vi "OpenMultipleDevices.vi"() -> ()   [LabVIEW 2013]
uses:
  C:/Code/Apps/Utilities/AG-UC2-UC8/AG-UC2-UC8/Install/Samples/LabVIEW/LabVIEW 2013/CmdLibAgilis.dll
  CmdLibAgilis.dll
panel:
  in  "FwVersion":string
  out "Output:":string
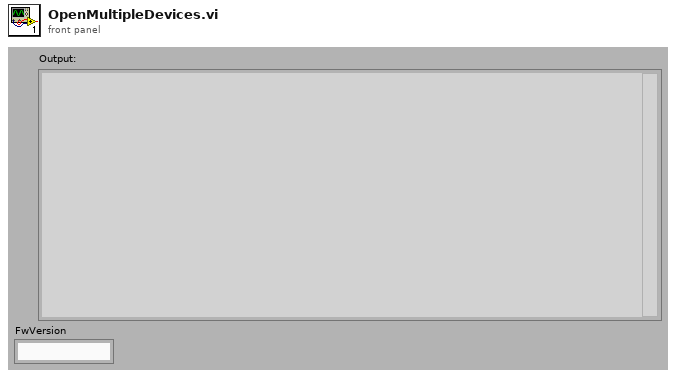
[diagram p1: front panel]
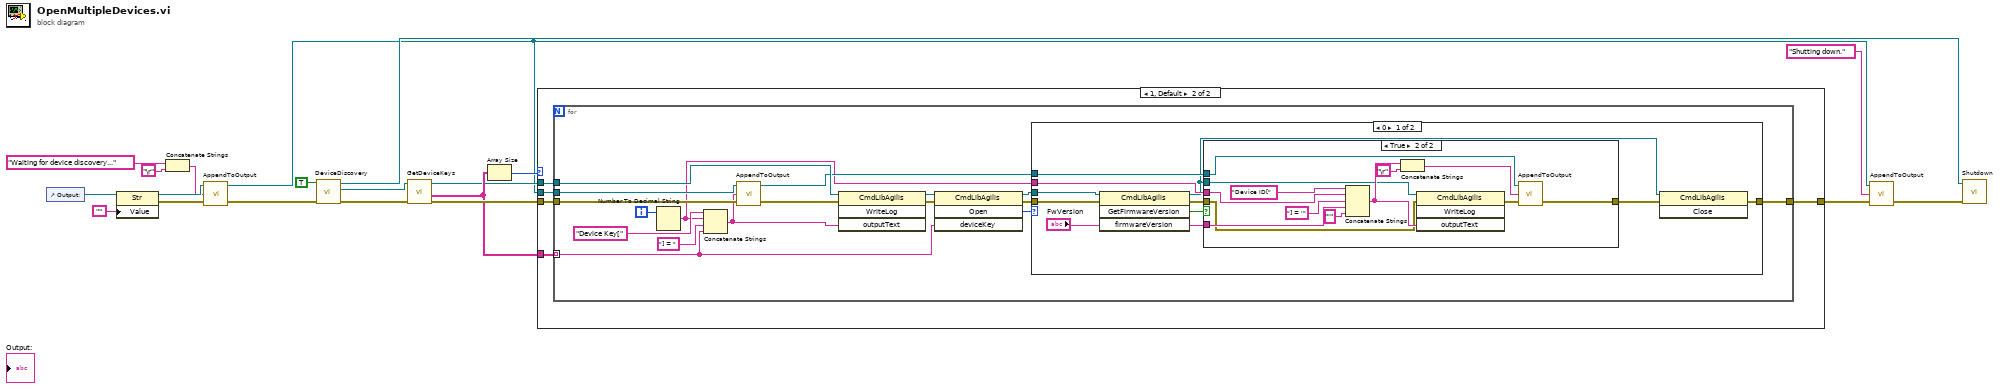
[diagram p0: block diagram]
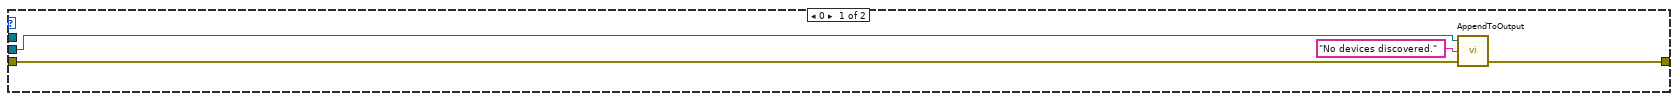
[diagram p2: hidden frame]
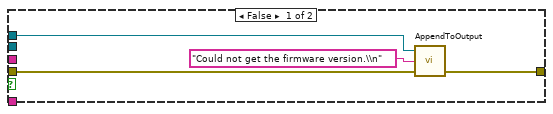
[diagram p3: hidden frame]
diagram:
  n1 = control-ref of="Output:"() -> (w20:refnum<vi>)
  n2 = property class="Str"(reference=w20, "Value"="") -> (reference out=w17:refnum<vi>, error out=w18:errorcluster)  [unwired: 1 in]
  n3 = Concatenate Strings("Waiting for device discovery...", "\r") -> (w7:string)
  n4 = call "AppendToOutput.vi"("error in"=w18, "Input String"=w7, "Output Refnum In"=w17) -> ("error out"=w15:errorcluster, "Output Refnum Out"=w1:refnum<vi>)  [unwired: 1 in]
  n5 = call "DeviceDiscovery.vi"("error in (no error)"=w15, "logging"=TRUE) -> ("error out"=w14:errorcluster, "CmdLib Out"=w13:refnum<k24>, "VCPIOLib Out"=w10:refnum<k24>)  [unwired: 3 in]
  n6 = call "GetDeviceKeys.vi"("error in (no error)"=w14, "CmdLib In"=w13) -> ("error out"=w11:errorcluster, "Device Keys"=w9:string[], "CmdLib Out"=w8:refnum<k24>)  [unwired: 3 in]
  n7 = Array Size(array=w9) -> (size(s)=w12:i32)
  n8 = case shown="1, Default" w12 {
    tunnel: w1 -> [w24 w28]
    tunnel: w11 -> [w23 w27]
    tunnel: w9 -> [_ w29]
    tunnel: w8 -> [_ w26]
    tunnel: [w21 w25] -> w2
    frame 0 {
      n9 = call "AppendToOutput.vi"("error in"=w23, "Input String"="No devices discovered.", "Output Refnum In"=w24) -> ("error out"=w21:errorcluster)  [unwired: 1 in, 1 out]
    }
    frame 1, Default {
      n10 = for {
        tunnel: w29 -> [w38] mode=indexing
        tunnel: w28 -> [w43]
        tunnel: w27 -> [w42]
        tunnel: w26 -> [w39]
        tunnel: [w31] -> w25
        i -> [w46]
        n11 = Number To Decimal String(number=w46) -> (decimal integer string=w30:string)  [unwired: 1 in]
        n12 = Concatenate Strings("Device Key[", w30, "] = ", w38) -> (w41:string)
        n13 = call "AppendToOutput.vi"("error in"=w42, "Input String"=w41, "Output Refnum In"=w43) -> ("error out"=w40:errorcluster, "Output Refnum Out"=w32:refnum<vi>)  [unwired: 1 in]
        n14 = invoke class="CmdLibAgilis" method="WriteLog"(reference=w39, error in=w40, "outputText"=w41) -> (reference out=w37:refnum<k24>, error out=w36:errorcluster)  [unwired: 1 in, 2 out]
        n15 = invoke class="CmdLibAgilis" method="Open"(reference=w37, error in=w36, "deviceKey"=w38) -> (reference out=w34:refnum<k24>, error out=w33:errorcluster, "Open"=w35:i32)  [unwired: 1 in, 1 out]
        n16 = case shown="0" w35 {
          tunnel: w34 -> [w57 _]
          tunnel: w33 -> [w56 w75]
          tunnel: w32 -> [w52 _]
          tunnel: [w50 w75] -> w31
          tunnel: w30 -> [w48 _]
          frame 0 {
            n17 = invoke class="CmdLibAgilis" method="GetFirmwareVersion"(reference=w57, error in=w56, "firmwareVersion"="FwVersion") -> (reference out=w47:refnum<k24>, error out=w53:errorcluster, "GetFirmwareVersion"=w54:bool, "firmwareVersion"=w49:string)  [unwired: 1 in]
            n18 = case shown="True" w54 {
              tunnel: w53 -> [w61 w66]
              tunnel: w52 -> [w60 w69]
              tunnel: [w58 w64] -> w51
              tunnel: w49 -> [_ w72]
              tunnel: w48 -> [_ w71]
              tunnel: w47 -> [_ w63]
              frame False {
                n19 = call "AppendToOutput.vi"("error in"=w61, "Input String"="Could not get the firmware version.\\n" ("firmwareVersion"), "Output Refnum In"=w60) -> ("error out"=w58:errorcluster)  [unwired: 1 in, 1 out]
              }
              frame True {
                n20 = Concatenate Strings("Device ID[", w71, "] = '", w72, "'" ("string")) -> (w68:string)
                n21 = Concatenate Strings(w68, "\r") -> (w67:string)
                n22 = invoke class="CmdLibAgilis" method="WriteLog"(reference=w63, error in=w66, "outputText"=w68) -> (error out=w65:errorcluster)  [unwired: 1 in, 3 out]
                n23 = call "AppendToOutput.vi"("error in"=w65, "Input String"=w67, "Output Refnum In"=w69) -> ("error out"=w64:errorcluster)  [unwired: 1 in, 1 out]
              }
            }
            n24 = invoke class="CmdLibAgilis" method="Close"(reference=w47, error in=w51) -> (error out=w50:errorcluster)  [unwired: 1 in, 2 out]
          }
          frame 1, Default {
          }
        }
      }
    }
  }
  n25 = call "AppendToOutput.vi"("error in"=w2, "Input String"="Shutting down." ("concatenated string"), "Output Refnum In"=w1) -> ("error out"=w3:errorcluster)  [unwired: 1 in, 1 out]
  n26 = call "Shutdown.vi"("error in (no error)"=w3, "VCPIOLib In"=w10) -> ()  [unwired: 9 in, 1 out]
